vi "Rotation2d_GetTan.vi"(11 "in ROTATION":T1={"VALUE"=0.0, "COS"=1.0, "SIN"=0.0} {"SIN" format="%13.4f"; "COS" format="%13.4f"; "VALUE" format="%13.4f"}) -> (3 "Tangent":dbl)   [LabVIEW 2019, in "Trajectory_Library.lvlib"]
doc: "Returns the tanget of the rotation.\n\nParameters:\n - in ROTATION - This ROTATION data structure\n\nReturns:a\n - Tangent of the ROTATAION"
uses:
  Trajectory_Library.lvlib
  TypeDef/ROTATION2D.ctl
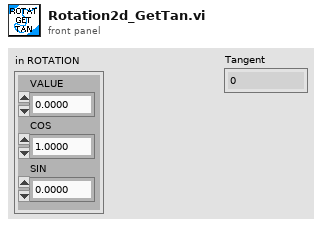
[diagram p1: front panel]
types:
  T1 = typedef "Trajectory_Library.lvlib/ROTATION2D.ctl" = cluster{"VALUE":dbl, "COS":dbl, "SIN":dbl}
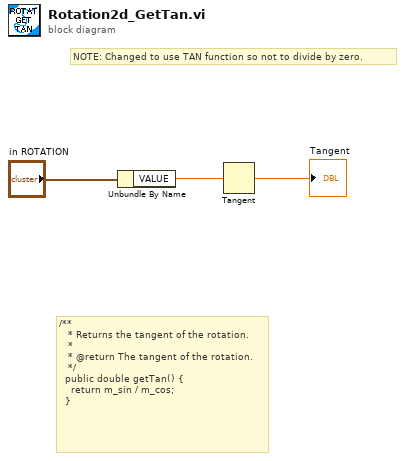
[diagram p0: block diagram]
diagram:
  # "NOTE: Changed to use TAN function so not to divide by zero."
  # "/**\n   * Returns the tangent of the rotation.\n   *\n   * @return The tangent of the rotation.\n   */\n  public double getTan() {\n    return m_sin / m_cos;\n  }"
  n1 = Unbundle By Name("in ROTATION") -> ("VALUE"=w2:dbl)
  n2 = Tangent(1:w2) -> (0:→"Tangent":dbl)
